vi "Shutdown Core.vi"(8 "error in (no error)":errorcluster, 11 "NI-SWITCH Consumer in":refnum<class "NI-SWITCH Consumer.lvclass">) -> (0 "error out":errorcluster, 3 "NI-SWITCH Consumer out":refnum<class "NI-SWITCH Consumer.lvclass">)   [LabVIEW 2020, in "NI-SWITCH Messaging.lvlib" / "NI-SWITCH Consumer.lvclass"]
uses:
  NI-SWITCH Consumer.lvclass
  NI-SWITCH Consumer.lvclass/NI-SWITCH Consumer.ctl
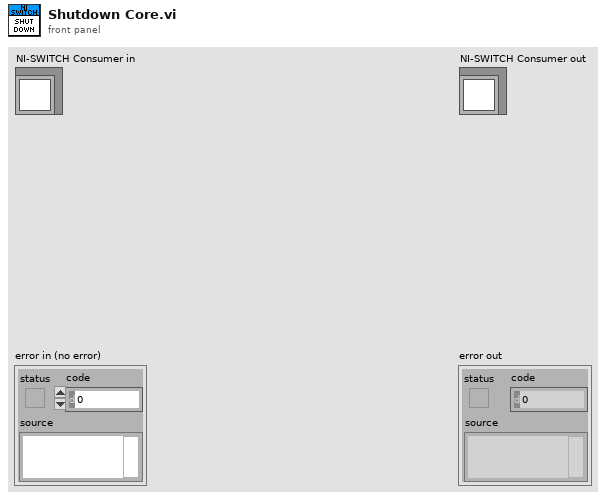
[diagram p1: front panel]
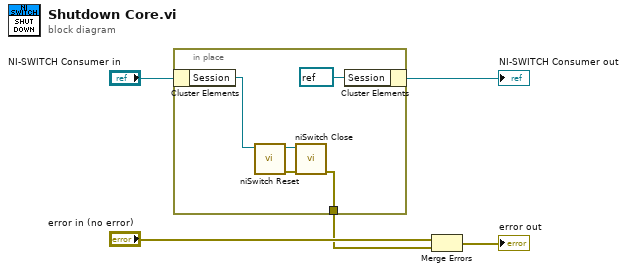
[diagram p0: block diagram]
diagram:
  n1 = in-place {
    in-place-border: [w10] -> w3
    n2 = in-place-cluster #1("NI-SWITCH Consumer in") -> ("Session"=w9:refnum<k15>)
    n3 = call <instrlib>:"niSwitch Reset.vi"("instrument handle"=w9) -> ("error out"=w7:errorcluster, "instrument handle out"=w8:refnum<k15>)  [unwired: 9 in]
    n4 = call <instrlib>:"niSwitch Close.vi"("error in (no error)"=w7, "instrument handle"=w8) -> ("error out"=w10:errorcluster)  [unwired: 9 in]
    n5 = in-place-cluster #1("Session"=refnum<k15> refnum) -> (→"NI-SWITCH Consumer out":refnum<class "NI-SWITCH Consumer.lvclass">)
  }
  n6 = Merge Errors("error in (no error)", w3) -> (→"error out":errorcluster)
